vi "SIM_CurrentOutput.vi"(11 "zin (m)":dbl) -> (3 "Current Out (A)":dbl)   [LabVIEW 2019]
uses:
  <vilib>/ptbypt/NI_PtbyPt.lvlib
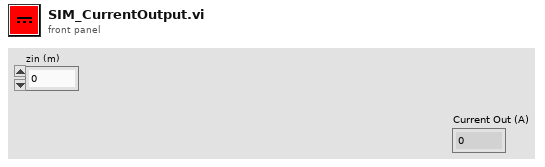
[diagram p1: front panel]
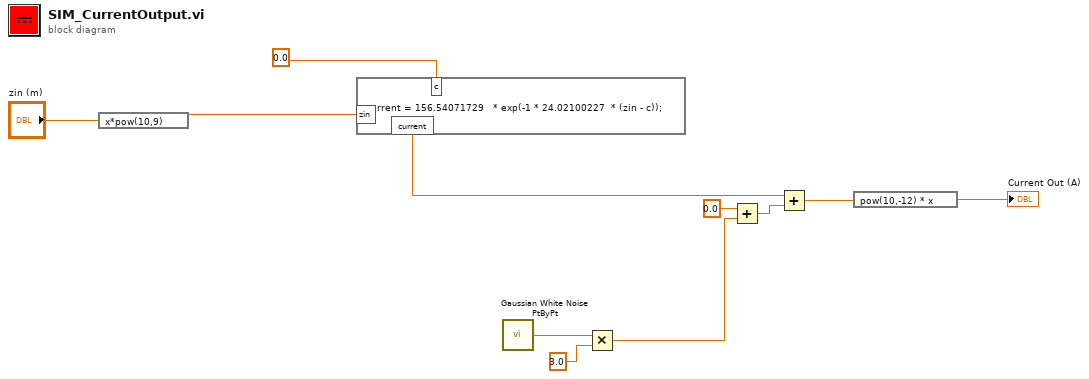
[diagram p0: block diagram]
diagram:
  n1 = expression code="x*pow(10,9)"("zin (m)") -> (w2:dbl)
  n2 = formula code="current = 156.54071729   * exp(-1 * 24.02100227  * (zin - c));"("zin"=w2, "c"=0.0 ("Zread")) -> ("current"=w6:dbl)
  n3 = call <vilib>:"Gaussian White Noise PtByPt.vi"() -> ("Gaussian white noise"=w11:dbl)  [unwired: 3 in]
  n4 = Multiply(x=w11, y=3.0) -> (x*y=w8:dbl)
  n5 = Add(x=0.0, y=w8) -> (x+y=w9:dbl)
  n6 = Add(x=w6, y=w9) -> (x+y=w5:dbl)
  n7 = expression code="pow(10,-12) * x"(w5) -> (→"Current Out (A)":dbl)
